vi "2 RudderControlPI.vi"(9 "use PID?":bool=TRUE, 10 "Desired Heading":dbl) -> (2 "Rudder Output":dbl)   [LabVIEW 2011]
uses:
  2 Typedefs/PI Constants.ctl
  2 Globals/2 Global.vi
  2 Globals/2 TuningConstants.vi
  <vilib>/addons/control/pid/NI_PID_pid.lvlib
  <vilib>/addons/control/pid/pid.llb/PID (DBL).vi
  <vilib>/ptbypt/NI_PtbyPt.lvlib
  <vilib>/addons/control/pid/NI_PID_autopid.lvlib
panel:
  out "Boolean 2":bool
  out "Boolean":bool
  out "PID gains out":T1={"proportional gain (Kc)"=1.0, "integral time (Ti, min)"=0.01, "derivative time (Td, min)"=0.0} {"derivative time (Td, min)" format="%.3f"; "integral time (Ti, min)" format="%.3f"; "proportional gain (Kc)" format="%.3f"}
  out "tuning completed?":bool
  in  "autotuning parameters":T2={"controller type"=1, "relay cycles"=3, "relay amplitude"=1.0, "control specification"=2, "PV noise level"=0.1} {"PV noise level" format="%.2f"; "control specification" items=["normal", "fast", "slow"]; "relay amplitude" format="%.2f"; "controller type" items=["PID", "PI", "P"]}
  in  "autotune? (F)":bool
  out "PID State":dbl format="%0.2f"
  out "PID setpoint":dbl
  out "PI Constants":T3={"Proportional Gain"=5000.0, "Integral Time"=0.2, "Derivative Time"=0.1}
  in  "Maximum Rudder":dbl=40.0
  out "Current Heading":dbl
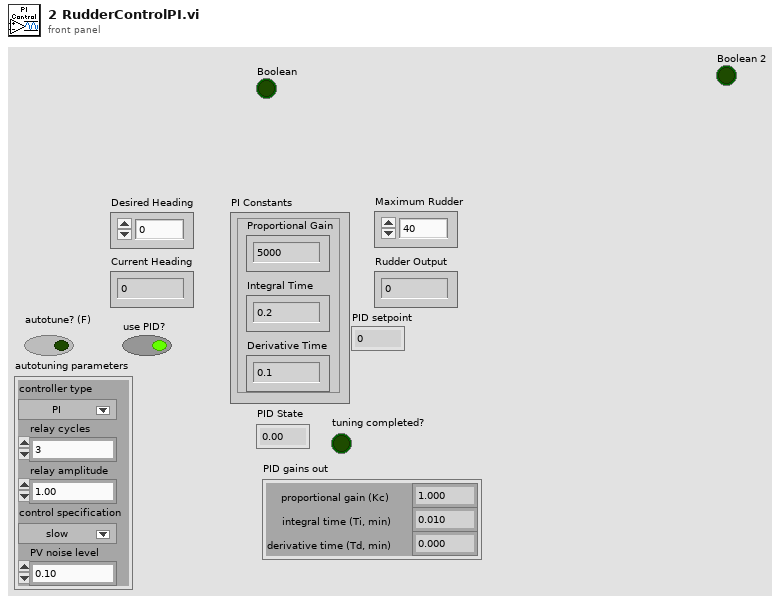
[diagram p1: front panel]
types:
  T1 = cluster{"proportional gain (Kc)":dbl, "integral time (Ti, min)":dbl, "derivative time (Td, min)":dbl}
  T2 = cluster{"controller type":u16, "relay cycles":i32, "relay amplitude":dbl, "control specification":u16, "PV noise level":dbl}
  T3 = typedef "PI Constants.ctl" = cluster{"Proportional Gain":dbl, "Integral Time":dbl, "Derivative Time":dbl}
  T4 = typedef "heading.ctl" = dbl
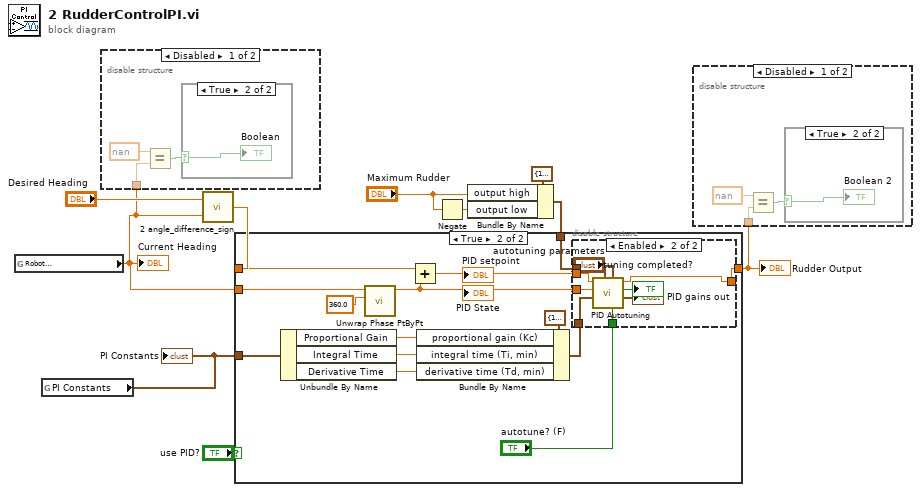
[diagram p0: block diagram]
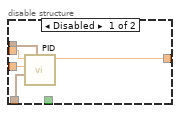
[diagram p7: hidden frame]
diagram:
  n1 = global read "2 Global.vi" "Robot\nHeading"() -> (w2:T4)
  "Current Heading" <- w2
  n2 = global read "2 TuningConstants.vi" "PI Constants"() -> (w4:T3)
  "PI Constants" <- w4
  n3 = disable-structure shown="Disabled" {
    disable-tunnel: w2 -> [w13 _]
    frame Disabled {
      n4 = Equal?(x=nan, y=w13) -> (x = y?=w11:bool)
      n5 = case shown="True" w11 {
        selector: w11 -> [_ w14]
        frame False {
        }
        frame True {
          "Boolean" <- w14
        }
      }
    }
    frame Enabled {
    }
  }
  n6 = call "2 angle_difference_sign.vi"("Angle 2"=w2, "Angle 1"="Desired Heading") -> ("Difference"=w10:dbl)
  n7 = Negate(x="Maximum Rudder") -> (-x=w8:dbl)
  n8 = Bundle By Name(cluster=cluster{"output high":dbl, "output low":dbl} {"output high"=100.0, "output low"=-100.0} ("output range"), "output high"="Maximum Rudder", "output low"=w8) -> (w5:cluster{"output high":dbl, "output low":dbl})
  n9 = case shown="True" "use PID?" {
    tunnel: w10 -> [w15 w20]
    tunnel: w4 -> [_ w27]
    tunnel: w5 -> [_ w29]
    tunnel: w2 -> [_ w21]
    tunnel: [w15 w17] -> w1
    frame False {
    }
    frame True {
      n10 = Unbundle By Name(w27) -> ("Proportional Gain"=w25:dbl, "Integral Time"=w24:dbl, "Derivative Time"=w23:dbl)
      n11 = call <vilib>:"Unwrap Phase PtByPt.vi"("wrap base"=360.0, "phase"=w21) -> ("unwrapped phase"=w19:dbl)  [unwired: 9 in]
      "PID State" <- w19
      n12 = Add(x=w20, y=w19) -> (x+y=w18:dbl)
      "PID setpoint" <- w18
      n13 = Bundle By Name(cluster=T1 {"proportional gain (Kc)"=1.0, "integral time (Ti, min)"=0.01, "derivative time (Td, min)"=0.0} ("PID gains"), "proportional gain (Kc)"=w25, "integral time (Ti, min)"=w24, "derivative time (Td, min)"=w23) -> (w26:T1)
      n14 = disable-structure shown="Enabled" {
        disable-tunnel: w29 -> [w34 w39]
        disable-tunnel: w26 -> [w33 w41]
        disable-tunnel: w19 -> [w32 w42]
        disable-tunnel: w18 -> [w31 w43]
        disable-tunnel: [w30 w35] -> w17
        disable-tunnel: "autotune? (F)" -> [_ w40]
        frame Disabled {
          n15 = call-poly <vilib>:"PID.vi"("output range"=w34, "PID gains"=w33, "process variable"=w32, "setpoint"=w31) -> ("output"=w30:dbl)  [unwired: 6 in, 1 out]
        }
        frame Enabled {
          n16 = call <vilib>:"PID Autotuning.vi"("autotune? (F)"=w40, "autotuning parameters"="autotuning parameters", "output range"=w39, "PID gains"=w41, "process variable"=w42, "setpoint"=w43) -> ("PID gains out"=→"PID gains out":T1, "tuning completed?"=→"tuning completed?":bool, "output"=w35:dbl)  [unwired: 2 in, 1 out]
        }
      }
    }
  }
  "Rudder Output" <- w1
  n17 = disable-structure shown="Disabled" {
    disable-tunnel: w1 -> [w44 _]
    frame Disabled {
      n18 = Equal?(x=nan, y=w44) -> (x = y?=w46:bool)
      n19 = case shown="True" w46 {
        selector: w46 -> [_ w47]
        frame False {
        }
        frame True {
          "Boolean 2" <- w47
        }
      }
    }
    frame Enabled {
    }
  }
